vi "Simple TCP - 사인파,삼각파Client.vi"() -> ()   [LabVIEW 2018]
doc: "Demonstrates how to open a connection to an TCP server, read the data being sent, and display the data on a chart. This VI is designed to stop if the TCP connection is terminated."
panel:
  out "웨이브폼 그래프":dynamicdata(graph)
  in  "Server Closed":string="The server VI closed the connection."
  in  "Stop":bool
  # "Overview: Demonstrates the use of the TCP functions to connect to a TCP server VI and receive data.\nInstructions:\n1. Ensure Simple TCP - Server.vi is already running.\n2. Run the VI.\n3. Click Stop to stop the VI. Note that if you stop the server VI, this VI will stop automatically."
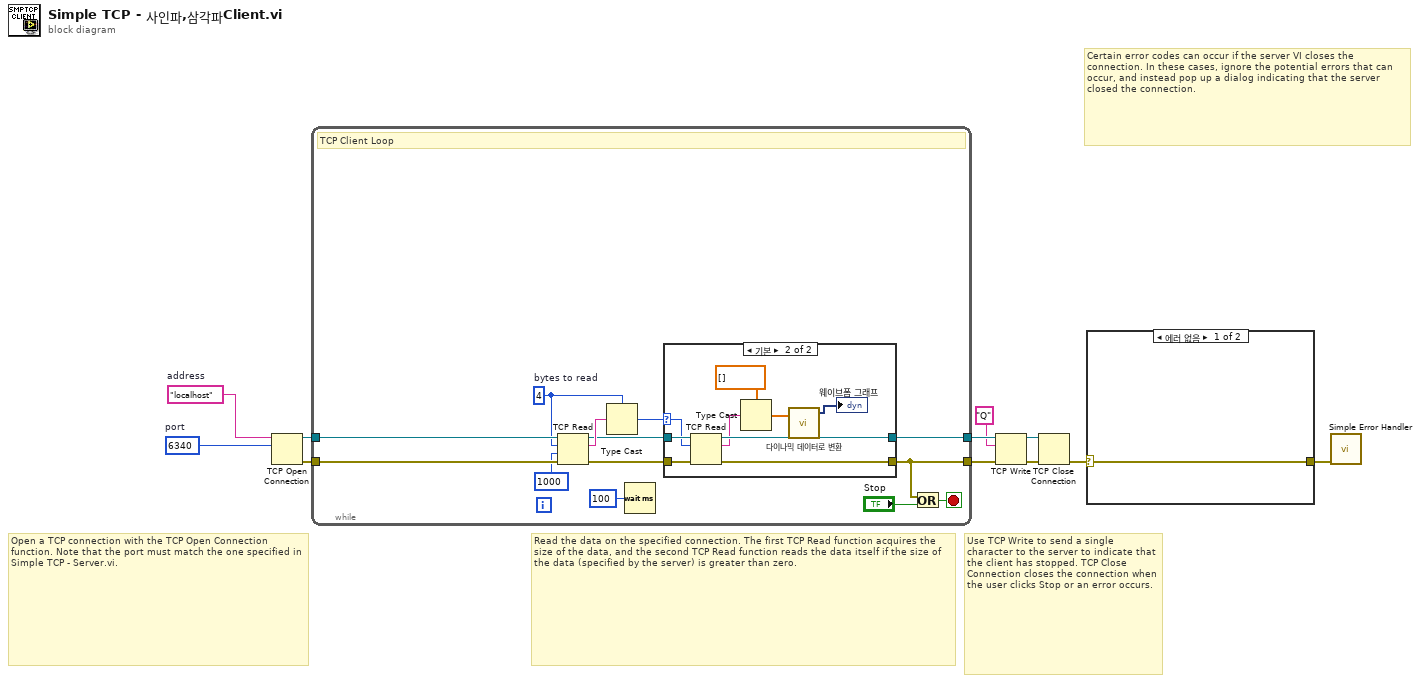
[diagram p0: block diagram]
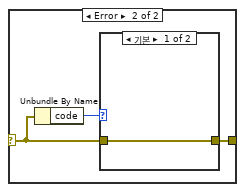
[diagram p2: hidden frame]
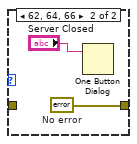
[diagram p3: hidden frame]
diagram:
  w1 = u16 6340  # port
  w2 = "localhost"  # address
  # "Certain error codes can occur if the server VI closes the connection. In these cases, ignore the potential errors that can occur, and instead pop up a dialog indicating that the server closed the connection."
  # "Use TCP Write to send a single character to the server to indicate that the client has stopped. TCP Close Connection closes the connection when the user clicks Stop or an error occurs."
  # "Read the data on the specified connection. The first TCP Read function acquires the size of the data, and the second TCP Read function reads the data itself if the size of the data (specified by the server) is greater than zero."
  # "Open a TCP connection with the TCP Open Connection function. Note that the port must match the one specified in Simple TCP - Server.vi."
  n1 = TCP Open Connection(address=w2, remote port or service name=w1) -> (connection ID=w11:refnum<k5>, error out=w10:errorcluster)  [unwired: 3 in]
  n2 = while {
    tunnel: w10 -> [w20]
    tunnel: w11 -> [w21]
    tunnel: [w15] -> w8
    tunnel: [w14] -> w6
    stop <- w17 stop-if-true
    w19 = 4  # bytes to read
    # "TCP Client Loop"
    n3 = TCP Read(connection ID=w21, bytes to read=w19, error in (no error)=w20, 9:1000 ("timeout ms (25000)")) -> (connection ID out=w23:refnum<k5>, data out=w24:string, error out=w22:errorcluster)  [unwired: 1 in]
    n4 = Type Cast(type=w19, x=w24) -> (*(type *) &x=w13:i32)
    n5 = Wait (ms)(milliseconds to wait=u32 100) -> ()  [unwired: 1 out]
    n6 = case shown="기본" w13 {
      selector: w13 -> [_ w29]
      tunnel: w23 -> [w26 w35]
      tunnel: w22 -> [w25 w34]
      tunnel: [w26 w32] -> w15
      tunnel: [w25 w31] -> w14
      frame ..0 {
        # "The server has not written any data"
      }
      frame Default {
        n7 = TCP Read(connection ID=w35, bytes to read=w29, error in (no error)=w34) -> (connection ID out=w32:refnum<k5>, data out=w30:string, error out=w31:errorcluster)  [unwired: 2 in]
        n8 = Type Cast(type=dbl[] [] ("chart"), x=w30) -> (*(type *) &x=w28:dbl[])
        n9 = call "다이나믹 데이터로 변환"("Array"=w28) -> ("Dynamic Data Type"=→"웨이브폼 그래프":dynamicdata)  [unwired: 3 in]
      }
    }
    n10 = Or(x=w14, y="Stop") -> (x .or. y?=w17:bool)
  }
  n11 = TCP Write(connection ID=w8, data in="Q", error in (no error)=w6) -> (connection ID out=w9:refnum<k5>, error out=w7:errorcluster)  [unwired: 2 out]
  n12 = TCP Close Connection(connection ID=w9, error in (no error)=w7) -> (error out=w4:errorcluster)  [unwired: 1 in, 1 out]
  n13 = case shown="에러 없음" w4 {
    selector: w4 -> [w36 w38]
    tunnel: [w36 w37] -> w3
    frame No Error {
    }
    frame Error {
      n14 = Unbundle By Name(w38) -> ("code"=w39:i32)
      n15 = case shown="기본" w39 {
        tunnel: w38 -> [w40 _]
        tunnel: [w40 w42] -> w37
        frame Default {
        }
        frame 62, 64, 66 {
          w42 = errorcluster {"status"=FALSE, "code"=0, "source"=""}  # No error
          n16 = One Button Dialog(message="Server Closed") -> ()  [unwired: 1 in, 1 out]
        }
      }
    }
  }
  n17 = call <vilib>:"Simple Error Handler.vi"("error in (no error)"=w3) -> ()  [unwired: 4 in, 5 out]
